vi "Init Buffer.vi"(8 "Error in":errorcluster, 11 "Async State Vars":T1) -> (0 "Error out":errorcluster, 3 "Async State Vars out":T1)   [LabVIEW 2020, in "Waveform-Processing-Custom-Device Engine.lvlib"]
uses:
  Waveform-Processing-Custom-Device Engine.lvlib
  <userlib>/Circular Buffer/Controls/Circular Buffer Operations.ctl
  <userlib>/Circular Buffer/Instance VIs/Circular Buffer(2D DBL).vi
  <vilib>/NI VeriStand/Custom Device Waveform API/Single Waveform Read (DBL)/Single Waveform Read (DBL).lvclass
  <vilib>/NI VeriStand/Custom Device Waveform API/Single Waveform Write (DBL)/Single Waveform Write (DBL).lvclass
  <vilib>/NI VeriStand/Custom Device API/Waveform Data Reference.ctl
  <vilib>/NI VeriStand/Custom Device API/Custom Device API.lvlib
  Types/AsyncStateVariables.ctl
  <vilib>/NI/NIVS Inline Async API/_Data Access Engine/Access Type Classes/Read/Read.lvclass
  <vilib>/NI/NIVS Inline Async API/_Data Access Engine/Data Access Engine/Types/Read.DVR.ctl
  <vilib>/NI/NIVS Inline Async API/_Data Access Engine/Data Access Engine/Data Access Engine.lvclass
  <vilib>/NI/NIVS Inline Async API/_Data Access Engine/Access Type Classes/Write/Write.lvclass
  <vilib>/NI/NIVS Inline Async API/_Data Access Engine/Data Access Engine/Types/Write.DVR.ctl
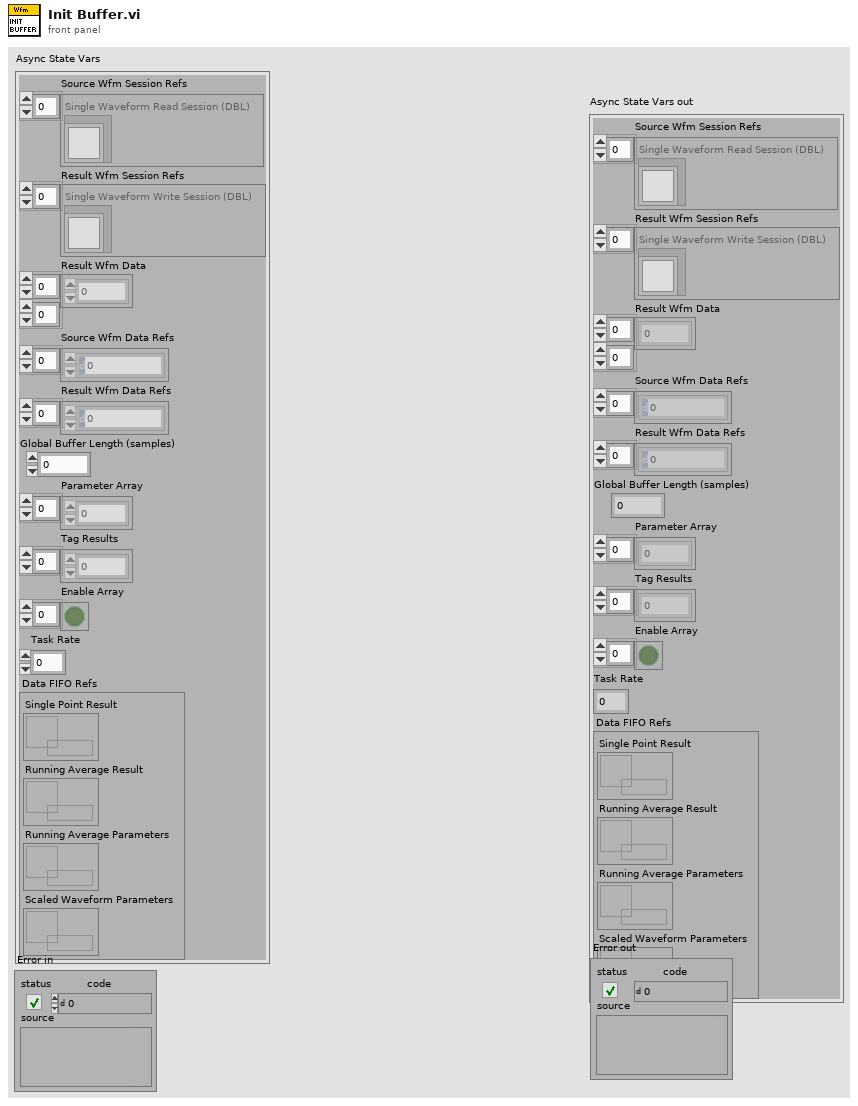
[diagram p1: front panel]
types:
  T1 = typedef "Waveform-Processing-Custom-Device Engine.lvlib/AsyncStateVariables.ctl" = cluster{"Source Wfm Session Refs":refnum<class "Single Waveform Read (DBL).lvclass">[], "Result Wfm Session Refs":refnum<class "Single Waveform Write (DBL).lvclass">[], "Result Wfm Data":dbl[][], "Source Wfm Data Refs":T2[], "Result Wfm Data Refs":T2[], "Global Buffer Length (samples)":dbl, "Parameter Array":dbl[], "Tag Results":dbl[], "Enable Array":bool[], "Task Rate":dbl, "Data FIFO Refs":cluster{"Single Point Result":T3, "Running Average Result":T3, "Running Average Parameters":T4, "Scaled Waveform Parameters":T4}}
  T2 = typedef "Custom Device API.lvlib/Waveform Data Reference.ctl" = i32
  T3 = typedef "Data Access Engine.lvlib/Data Access Engine.lvclass/Write.DVR.ctl" = refnum<data-value>
  T4 = typedef "Data Access Engine.lvlib/Data Access Engine.lvclass/Read.DVR.ctl" = refnum<data-value>
  T5 = typedef "Circular Buffer.lvlib/Circular Buffer Operations.ctl" = enum16{"Initialize", "Get Backlog", "Write", "Read (continuous)", "Read (most recent)"}
  T6 = cluster{"Samples per Channel":u32, "Channels":u32}
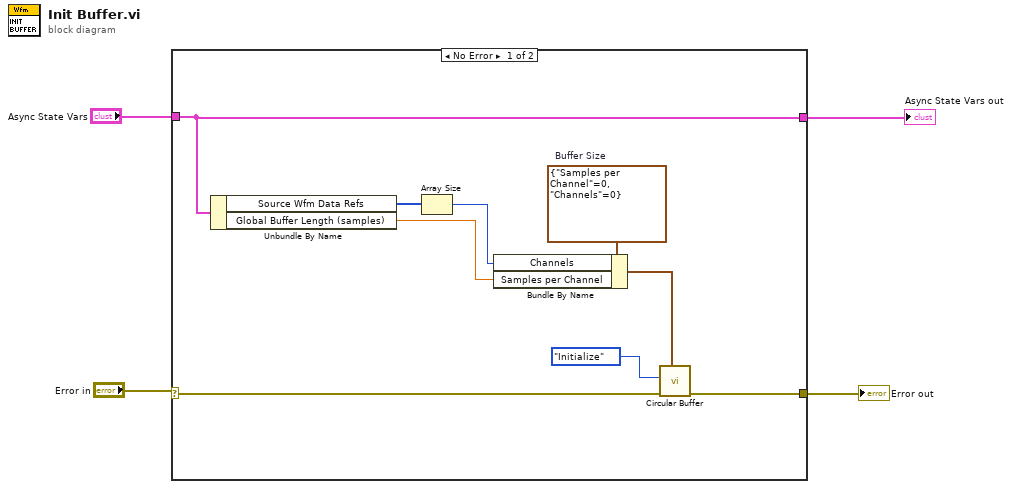
[diagram p0: block diagram]
diagram:
  n1 = case shown="No Error" "Error in" {
    selector: "Error in" -> [w13 w14]
    tunnel: "Async State Vars" -> [w5 w15]
    tunnel: [w12 w14] -> w2
    tunnel: [w5 w15] -> w1
    frame No Error {
      w9 = T6 {"Samples per Channel"=0, "Channels"=0}  # Buffer Size
      n2 = Unbundle By Name(w5) -> ("Source Wfm Data Refs"=w10:T2[], "Global Buffer Length (samples)"=w7:dbl)
      n3 = Array Size(array=w10) -> (size(s)=w8:i32)
      n4 = Bundle By Name(cluster=w9, "Channels"=w8, "Samples per Channel"=w7) -> (w6:T6)
      n5 = call-poly <userlib>:"Circular Buffer.vi"("Buffer Size"=w6, "error in (no error)"=w13, "Operation"=Circular_Buffer_Operations."Initialize") -> ("error out"=w12:errorcluster)  [unwired: 5 in, 3 out]
    }
    frame Error {
    }
  }
  "Async State Vars out" <- w1
  "Error out" <- w2
